vi "FPGA Read Indicator Array Address by Name.vi"(8 "error in (no error)":errorcluster, 9 "Name":string, 10 "Data Type":T1, 11 "FPGA Interface Base in":refnum<class "FPGA Interface Base.lvclass">) -> (0 "error out":errorcluster, 1 "Found?":bool, 2 "Address":u32, 3 "FPGA Interface Base out":refnum<class "FPGA Interface Base.lvclass">, 5 "Num Elements":u32)   [LabVIEW 2010, in "FPGA Interface Base.lvclass"]
uses:
  <userlib>/_FPGA Interface Advanced Tools/FPGA Interface Base/FPGA Interface Base.lvclass
  <vilib>/rvi/DataTransferAndStorage/Container/Common/niFpgaDataTypeControl.ctl
  <userlib>/_FPGA Interface Advanced Tools/FPGA Interface Base/FPGA Interface Base.lvclass/FPGA Interface Base.ctl
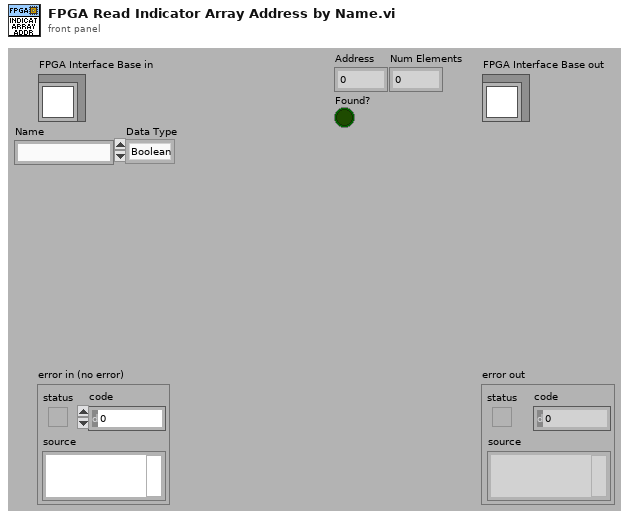
[diagram p1: front panel]
types:
  T1 = typedef "niFpgaDataTypeControl.ctl" = enum32{"Boolean", "I8", "I16", "I32", "I64", "U8", "U16", "U32", "U64", "FXP", "CustomControl"}
  T2 = typedef "FPGA Interface Base.lvclass/FPGA Session.ctl" = refnum<data-value>
  T3 = typedef "FPGA Interface Base.lvclass/FPGA Session Data.ctl" = cluster{"Session Out":u32, "Indicator Scalars":T4, "Indicator Arrays":T6, "Control Scalars":T4, "Control Arrays":T6, "TargetToHost FIFO Channels":T8, "HostToTarget FIFO Channels":T8, "All FIFOs":T9[], "IRQ Context Queue":refnum<queue>}
  T4 = typedef "FPGA Bitfile Utility.lvlib/Scalar Register Set.ctl" = cluster{"Boolean":T5[], "I8":T5[], "I16":T5[], "I32":T5[], "I64":T5[], "U8":T5[], "U16":T5[], "U32":T5[], "U64":T5[]}
  T5 = typedef "FPGA Bitfile Utility.lvlib/Scalar Register.ctl" = cluster{"Address":u32, "Name":string}
  T6 = typedef "FPGA Bitfile Utility.lvlib/Array Register Set.ctl" = cluster{"Boolean":T7[], "I8":T7[], "I16":T7[], "I32":T7[], "I64":T7[], "U8":T7[], "U16":T7[], "U32":T7[], "U64":T7[]}
  T7 = typedef "FPGA Bitfile Utility.lvlib/Array Register.ctl" = cluster{"Address":u32, "Num Elements":u32, "Name":string}
  T8 = typedef "FPGA Bitfile Utility.lvlib/FIFO Channel Set.ctl" = cluster{"Boolean":T9[], "I8":T9[], "I16":T9[], "I32":T9[], "I64":T9[], "U8":T9[], "U16":T9[], "U32":T9[], "U64":T9[]}
  T9 = typedef "FPGA Bitfile Utility.lvlib/FIFO Channel.ctl" = cluster{"Physical Channel":u32, "Name":string}
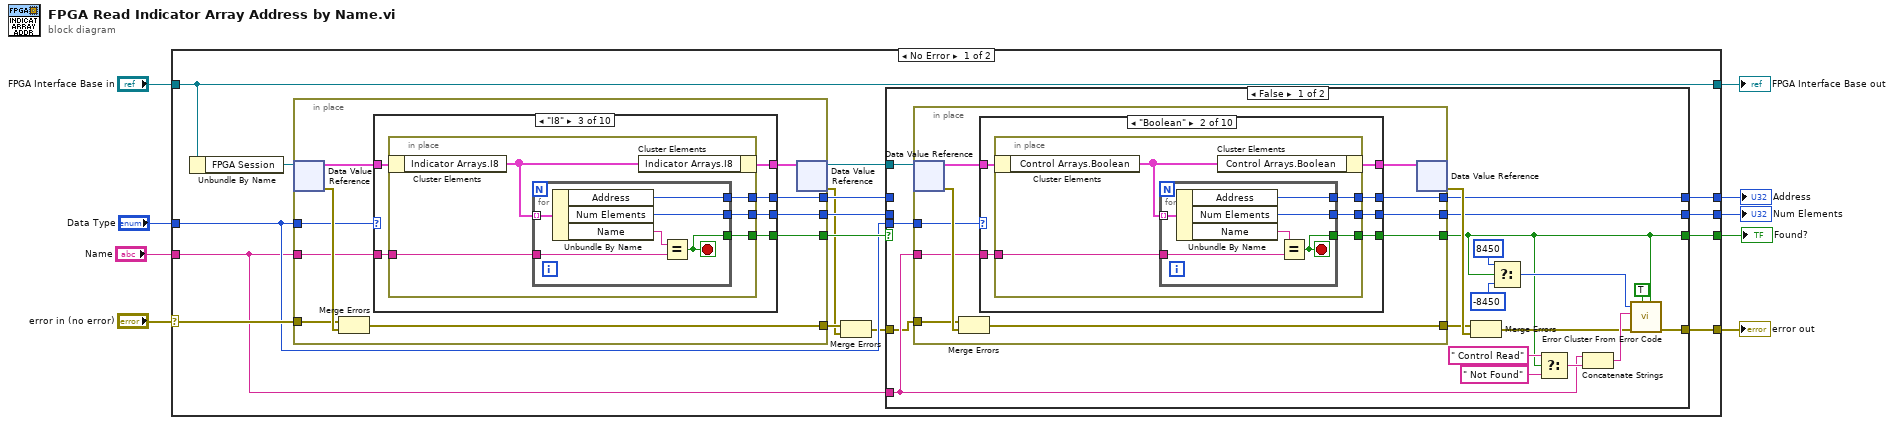
[diagram p0: block diagram]
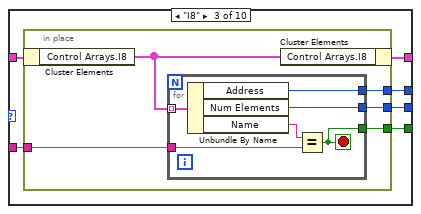
[diagram p3: hidden frame]
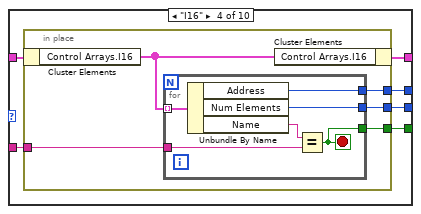
[diagram p4: hidden frame]
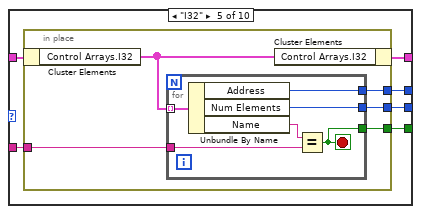
[diagram p5: hidden frame]
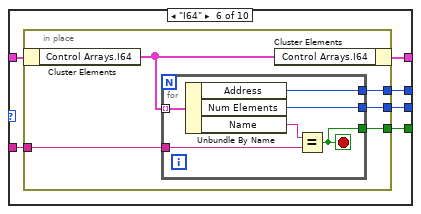
[diagram p6: hidden frame]
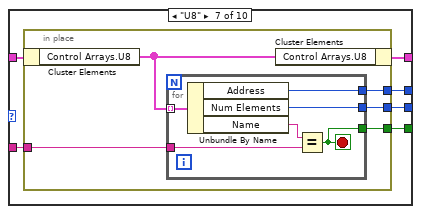
[diagram p7: hidden frame]
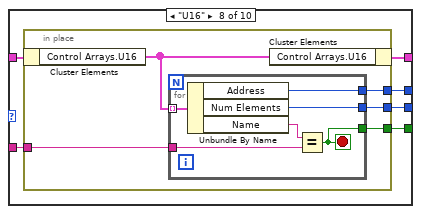
[diagram p8: hidden frame]
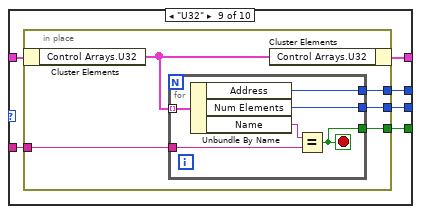
[diagram p9: hidden frame]
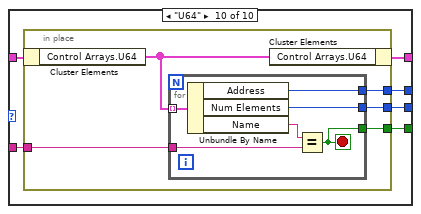
[diagram p10: hidden frame]
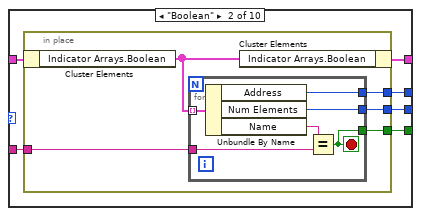
[diagram p13: hidden frame]
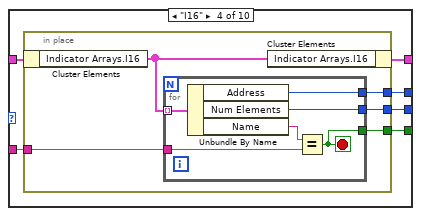
[diagram p14: hidden frame]
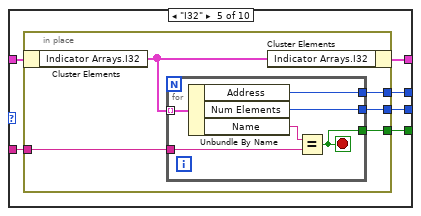
[diagram p15: hidden frame]
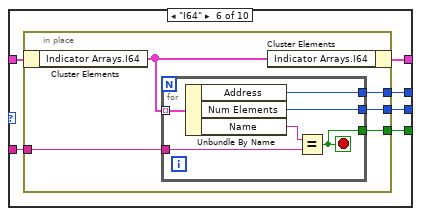
[diagram p16: hidden frame]
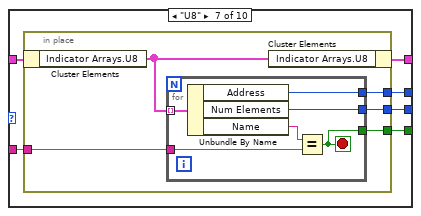
[diagram p17: hidden frame]
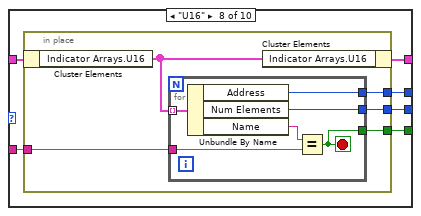
[diagram p18: hidden frame]
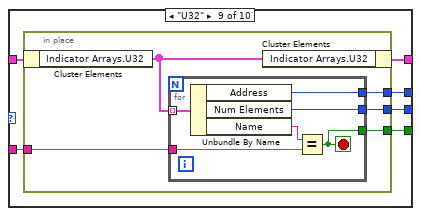
[diagram p19: hidden frame]
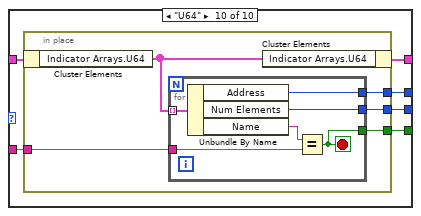
[diagram p20: hidden frame]
diagram:
  n1 = case shown="No Error" "error in (no error)" {
    selector: "error in (no error)" -> [w23 w377]
    tunnel: [w13 w377] -> w8
    tunnel: [w25 w378] -> w6
    tunnel: "FPGA Interface Base in" -> [w25 w378]
    tunnel: [w12 _] -> w5
    tunnel: [w11 _] -> w4
    tunnel: "Name" -> [w14 _]
    tunnel: "Data Type" -> [w18 _]
    tunnel: [w10 _] -> w1
    frame No Error {
      n2 = Unbundle By Name(w25) -> ("FPGA Session"=w24:T2)
      n3 = in-place {
        in-place-border: w14 -> [w219]
        in-place-border: [w218] -> w21
        in-place-border: [w217] -> w19
        in-place-border: [w216] -> w17
        in-place-border: w23 -> [w215]
        in-place-border: w18 -> [w214]
        in-place-border: [w213] -> w20
        n4 = in-place-dvr #1(w24) -> (w221:T3, w222:errorcluster)
        n5 = Merge Errors(w215, w222) -> (w216:errorcluster)
        n6 = case shown="\"I8\"" w214 {
          tunnel: w221 -> [w223 w229 w246 w263 w280 w297 w314 w331 w348 w365]
          tunnel: [w223 w228 w245 w262 w279 w296 w313 w330 w347 w364] -> w220
          tunnel: w219 -> [_ w227 w244 w261 w278 w295 w312 w329 w346 w363]
          tunnel: [_ w226 w243 w260 w277 w294 w311 w328 w345 w362] -> w218
          tunnel: [_ w225 w242 w259 w276 w293 w310 w327 w344 w361] -> w217
          tunnel: [_ w224 w241 w258 w275 w292 w309 w326 w343 w360] -> w213
          frame Default {
          }
          frame "Boolean" {
            n7 = in-place {
              in-place-border: w227 -> [w233]
              in-place-border: [w232] -> w226
              in-place-border: [w231] -> w225
              in-place-border: [w230] -> w224
              n8 = in-place-cluster #2(w229) -> ("Indicator Arrays.Boolean"=w234:T7[])
              n9 = for {
                tunnel: w234 -> [w240] mode=indexing
                tunnel: [w238] -> w232
                tunnel: [w237] -> w231
                tunnel: w233 -> [w236]
                tunnel: [w235] -> w230
                stop <- w237 stop-if-true
                n10 = Unbundle By Name(w240) -> ("Address"=w238:u32, "Num Elements"=w235:u32, "Name"=w239:string)
                n11 = Equal?(x=w239, y=w236) -> (x = y?=w237:bool)
              }
              n12 = in-place-cluster #2("Indicator Arrays.Boolean"=w234) -> (w228:T3)
            }
          }
          frame "I8" {
            n13 = in-place {
              in-place-border: w244 -> [w250]
              in-place-border: [w249] -> w243
              in-place-border: [w248] -> w242
              in-place-border: [w247] -> w241
              n14 = in-place-cluster #3(w246) -> ("Indicator Arrays.I8"=w251:T7[])
              n15 = for {
                tunnel: w251 -> [w257] mode=indexing
                tunnel: [w256] -> w249
                tunnel: [w255] -> w248
                tunnel: w250 -> [w254]
                tunnel: [w252] -> w247
                stop <- w255 stop-if-true
                n16 = Unbundle By Name(w257) -> ("Address"=w256:u32, "Num Elements"=w252:u32, "Name"=w253:string)
                n17 = Equal?(x=w253, y=w254) -> (x = y?=w255:bool)
              }
              n18 = in-place-cluster #3("Indicator Arrays.I8"=w251) -> (w245:T3)
            }
          }
          frame "I16" {
            n19 = in-place {
              in-place-border: w261 -> [w267]
              in-place-border: [w266] -> w260
              in-place-border: [w265] -> w259
              in-place-border: [w264] -> w258
              n20 = in-place-cluster #4(w263) -> ("Indicator Arrays.I16"=w268:T7[])
              n21 = for {
                tunnel: w268 -> [w274] mode=indexing
                tunnel: [w272] -> w266
                tunnel: [w271] -> w265
                tunnel: w267 -> [w270]
                tunnel: [w269] -> w264
                stop <- w271 stop-if-true
                n22 = Unbundle By Name(w274) -> ("Address"=w272:u32, "Num Elements"=w269:u32, "Name"=w273:string)
                n23 = Equal?(x=w273, y=w270) -> (x = y?=w271:bool)
              }
              n24 = in-place-cluster #4("Indicator Arrays.I16"=w268) -> (w262:T3)
            }
          }
          frame "I32" {
            n25 = in-place {
              in-place-border: w278 -> [w284]
              in-place-border: [w283] -> w277
              in-place-border: [w282] -> w276
              in-place-border: [w281] -> w275
              n26 = in-place-cluster #5(w280) -> ("Indicator Arrays.I32"=w285:T7[])
              n27 = for {
                tunnel: w285 -> [w291] mode=indexing
                tunnel: [w289] -> w283
                tunnel: [w288] -> w282
                tunnel: w284 -> [w287]
                tunnel: [w286] -> w281
                stop <- w288 stop-if-true
                n28 = Unbundle By Name(w291) -> ("Address"=w289:u32, "Num Elements"=w286:u32, "Name"=w290:string)
                n29 = Equal?(x=w290, y=w287) -> (x = y?=w288:bool)
              }
              n30 = in-place-cluster #5("Indicator Arrays.I32"=w285) -> (w279:T3)
            }
          }
          frame "I64" {
            n31 = in-place {
              in-place-border: w295 -> [w301]
              in-place-border: [w300] -> w294
              in-place-border: [w299] -> w293
              in-place-border: [w298] -> w292
              n32 = in-place-cluster #6(w297) -> ("Indicator Arrays.I64"=w302:T7[])
              n33 = for {
                tunnel: w302 -> [w308] mode=indexing
                tunnel: [w306] -> w300
                tunnel: [w305] -> w299
                tunnel: w301 -> [w304]
                tunnel: [w303] -> w298
                stop <- w305 stop-if-true
                n34 = Unbundle By Name(w308) -> ("Address"=w306:u32, "Num Elements"=w303:u32, "Name"=w307:string)
                n35 = Equal?(x=w307, y=w304) -> (x = y?=w305:bool)
              }
              n36 = in-place-cluster #6("Indicator Arrays.I64"=w302) -> (w296:T3)
            }
          }
          frame "U8" {
            n37 = in-place {
              in-place-border: w312 -> [w318]
              in-place-border: [w317] -> w311
              in-place-border: [w316] -> w310
              in-place-border: [w315] -> w309
              n38 = in-place-cluster #7(w314) -> ("Indicator Arrays.U8"=w319:T7[])
              n39 = for {
                tunnel: w319 -> [w325] mode=indexing
                tunnel: [w323] -> w317
                tunnel: [w322] -> w316
                tunnel: w318 -> [w321]
                tunnel: [w320] -> w315
                stop <- w322 stop-if-true
                n40 = Unbundle By Name(w325) -> ("Address"=w323:u32, "Num Elements"=w320:u32, "Name"=w324:string)
                n41 = Equal?(x=w324, y=w321) -> (x = y?=w322:bool)
              }
              n42 = in-place-cluster #7("Indicator Arrays.U8"=w319) -> (w313:T3)
            }
          }
          frame "U16" {
            n43 = in-place {
              in-place-border: w329 -> [w335]
              in-place-border: [w334] -> w328
              in-place-border: [w333] -> w327
              in-place-border: [w332] -> w326
              n44 = in-place-cluster #8(w331) -> ("Indicator Arrays.U16"=w336:T7[])
              n45 = for {
                tunnel: w336 -> [w342] mode=indexing
                tunnel: [w340] -> w334
                tunnel: [w339] -> w333
                tunnel: w335 -> [w338]
                tunnel: [w337] -> w332
                stop <- w339 stop-if-true
                n46 = Unbundle By Name(w342) -> ("Address"=w340:u32, "Num Elements"=w337:u32, "Name"=w341:string)
                n47 = Equal?(x=w341, y=w338) -> (x = y?=w339:bool)
              }
              n48 = in-place-cluster #8("Indicator Arrays.U16"=w336) -> (w330:T3)
            }
          }
          frame "U32" {
            n49 = in-place {
              in-place-border: w346 -> [w352]
              in-place-border: [w351] -> w345
              in-place-border: [w350] -> w344
              in-place-border: [w349] -> w343
              n50 = in-place-cluster #9(w348) -> ("Indicator Arrays.U32"=w353:T7[])
              n51 = for {
                tunnel: w353 -> [w359] mode=indexing
                tunnel: [w357] -> w351
                tunnel: [w356] -> w350
                tunnel: w352 -> [w355]
                tunnel: [w354] -> w349
                stop <- w356 stop-if-true
                n52 = Unbundle By Name(w359) -> ("Address"=w357:u32, "Num Elements"=w354:u32, "Name"=w358:string)
                n53 = Equal?(x=w358, y=w355) -> (x = y?=w356:bool)
              }
              n54 = in-place-cluster #9("Indicator Arrays.U32"=w353) -> (w347:T3)
            }
          }
          frame "U64" {
            n55 = in-place {
              in-place-border: w363 -> [w369]
              in-place-border: [w368] -> w362
              in-place-border: [w367] -> w361
              in-place-border: [w366] -> w360
              n56 = in-place-cluster #10(w365) -> ("Indicator Arrays.U64"=w370:T7[])
              n57 = for {
                tunnel: w370 -> [w376] mode=indexing
                tunnel: [w374] -> w368
                tunnel: [w373] -> w367
                tunnel: w369 -> [w372]
                tunnel: [w371] -> w366
                stop <- w373 stop-if-true
                n58 = Unbundle By Name(w376) -> ("Address"=w374:u32, "Num Elements"=w371:u32, "Name"=w375:string)
                n59 = Equal?(x=w375, y=w372) -> (x = y?=w373:bool)
              }
              n60 = in-place-cluster #10("Indicator Arrays.U64"=w370) -> (w364:T3)
            }
          }
        }
        n61 = in-place-dvr #1(w220) -> (w22:T2, w15:errorcluster)
      }
      n62 = Merge Errors(w17, w15) -> (w16:errorcluster)
      n63 = case shown="False" w19 {
        selector: w19 -> [_ w211]
        tunnel: w22 -> [w34 _]
        tunnel: w16 -> [w29 w210]
        tunnel: w21 -> [_ w212]
        tunnel: [w32 w212] -> w12
        tunnel: [w27 w211] -> w11
        tunnel: [w36 w210] -> w13
        tunnel: w14 -> [w30 _]
        tunnel: w18 -> [w31 _]
        tunnel: w20 -> [_ w209]
        tunnel: [w26 w209] -> w10
        frame False {
          n64 = in-place {
            in-place-border: w30 -> [w48]
            in-place-border: [w49] -> w32
            in-place-border: [w46] -> w27
            in-place-border: [w53] -> w28
            in-place-border: w29 -> [w52]
            in-place-border: w31 -> [w47]
            in-place-border: [w45] -> w26
            n65 = in-place-dvr #11(w34) -> (w51:T3, w54:errorcluster)
            n66 = Merge Errors(w52, w54) -> (w53:errorcluster)
            n67 = case shown="\"Boolean\"" w47 {
              tunnel: w51 -> [w55 w61 w78 w95 w112 w129 w146 w163 w180 w197]
              tunnel: [w55 w60 w77 w94 w111 w128 w145 w162 w179 w196] -> w50
              tunnel: w48 -> [_ w59 w76 w93 w110 w127 w144 w161 w178 w195]
              tunnel: [_ w58 w75 w92 w109 w126 w143 w160 w177 w194] -> w49
              tunnel: [_ w57 w74 w91 w108 w125 w142 w159 w176 w193] -> w46
              tunnel: [_ w56 w73 w90 w107 w124 w141 w158 w175 w192] -> w45
              frame Default {
              }
              frame "Boolean" {
                n68 = in-place {
                  in-place-border: w59 -> [w65]
                  in-place-border: [w64] -> w58
                  in-place-border: [w63] -> w57
                  in-place-border: [w62] -> w56
                  n69 = in-place-cluster #12(w61) -> ("Control Arrays.Boolean"=w66:T7[])
                  n70 = for {
                    tunnel: w66 -> [w72] mode=indexing
                    tunnel: [w70] -> w64
                    tunnel: [w69] -> w63
                    tunnel: w65 -> [w68]
                    tunnel: [w67] -> w62
                    stop <- w69 stop-if-true
                    n71 = Unbundle By Name(w72) -> ("Address"=w70:u32, "Num Elements"=w67:u32, "Name"=w71:string)
                    n72 = Equal?(x=w71, y=w68) -> (x = y?=w69:bool)
                  }
                  n73 = in-place-cluster #12("Control Arrays.Boolean"=w66) -> (w60:T3)
                }
              }
              frame "I8" {
                n74 = in-place {
                  in-place-border: w76 -> [w82]
                  in-place-border: [w81] -> w75
                  in-place-border: [w80] -> w74
                  in-place-border: [w79] -> w73
                  n75 = in-place-cluster #13(w78) -> ("Control Arrays.I8"=w83:T7[])
                  n76 = for {
                    tunnel: w83 -> [w89] mode=indexing
                    tunnel: [w88] -> w81
                    tunnel: [w87] -> w80
                    tunnel: w82 -> [w86]
                    tunnel: [w84] -> w79
                    stop <- w87 stop-if-true
                    n77 = Unbundle By Name(w89) -> ("Address"=w88:u32, "Num Elements"=w84:u32, "Name"=w85:string)
                    n78 = Equal?(x=w85, y=w86) -> (x = y?=w87:bool)
                  }
                  n79 = in-place-cluster #13("Control Arrays.I8"=w83) -> (w77:T3)
                }
              }
              frame "I16" {
                n80 = in-place {
                  in-place-border: w93 -> [w99]
                  in-place-border: [w98] -> w92
                  in-place-border: [w97] -> w91
                  in-place-border: [w96] -> w90
                  n81 = in-place-cluster #14(w95) -> ("Control Arrays.I16"=w100:T7[])
                  n82 = for {
                    tunnel: w100 -> [w106] mode=indexing
                    tunnel: [w104] -> w98
                    tunnel: [w103] -> w97
                    tunnel: w99 -> [w102]
                    tunnel: [w101] -> w96
                    stop <- w103 stop-if-true
                    n83 = Unbundle By Name(w106) -> ("Address"=w104:u32, "Num Elements"=w101:u32, "Name"=w105:string)
                    n84 = Equal?(x=w105, y=w102) -> (x = y?=w103:bool)
                  }
                  n85 = in-place-cluster #14("Control Arrays.I16"=w100) -> (w94:T3)
                }
              }
              frame "I32" {
                n86 = in-place {
                  in-place-border: w110 -> [w116]
                  in-place-border: [w115] -> w109
                  in-place-border: [w114] -> w108
                  in-place-border: [w113] -> w107
                  n87 = in-place-cluster #15(w112) -> ("Control Arrays.I32"=w117:T7[])
                  n88 = for {
                    tunnel: w117 -> [w123] mode=indexing
                    tunnel: [w121] -> w115
                    tunnel: [w120] -> w114
                    tunnel: w116 -> [w119]
                    tunnel: [w118] -> w113
                    stop <- w120 stop-if-true
                    n89 = Unbundle By Name(w123) -> ("Address"=w121:u32, "Num Elements"=w118:u32, "Name"=w122:string)
                    n90 = Equal?(x=w122, y=w119) -> (x = y?=w120:bool)
                  }
                  n91 = in-place-cluster #15("Control Arrays.I32"=w117) -> (w111:T3)
                }
              }
              frame "I64" {
                n92 = in-place {
                  in-place-border: w127 -> [w133]
                  in-place-border: [w132] -> w126
                  in-place-border: [w131] -> w125
                  in-place-border: [w130] -> w124
                  n93 = in-place-cluster #16(w129) -> ("Control Arrays.I64"=w134:T7[])
                  n94 = for {
                    tunnel: w134 -> [w140] mode=indexing
                    tunnel: [w138] -> w132
                    tunnel: [w137] -> w131
                    tunnel: w133 -> [w136]
                    tunnel: [w135] -> w130
                    stop <- w137 stop-if-true
                    n95 = Unbundle By Name(w140) -> ("Address"=w138:u32, "Num Elements"=w135:u32, "Name"=w139:string)
                    n96 = Equal?(x=w139, y=w136) -> (x = y?=w137:bool)
                  }
                  n97 = in-place-cluster #16("Control Arrays.I64"=w134) -> (w128:T3)
                }
              }
              frame "U8" {
                n98 = in-place {
                  in-place-border: w144 -> [w150]
                  in-place-border: [w149] -> w143
                  in-place-border: [w148] -> w142
                  in-place-border: [w147] -> w141
                  n99 = in-place-cluster #17(w146) -> ("Control Arrays.U8"=w151:T7[])
                  n100 = for {
                    tunnel: w151 -> [w157] mode=indexing
                    tunnel: [w155] -> w149
                    tunnel: [w154] -> w148
                    tunnel: w150 -> [w153]
                    tunnel: [w152] -> w147
                    stop <- w154 stop-if-true
                    n101 = Unbundle By Name(w157) -> ("Address"=w155:u32, "Num Elements"=w152:u32, "Name"=w156:string)
                    n102 = Equal?(x=w156, y=w153) -> (x = y?=w154:bool)
                  }
                  n103 = in-place-cluster #17("Control Arrays.U8"=w151) -> (w145:T3)
                }
              }
              frame "U16" {
                n104 = in-place {
                  in-place-border: w161 -> [w167]
                  in-place-border: [w166] -> w160
                  in-place-border: [w165] -> w159
                  in-place-border: [w164] -> w158
                  n105 = in-place-cluster #18(w163) -> ("Control Arrays.U16"=w168:T7[])
                  n106 = for {
                    tunnel: w168 -> [w174] mode=indexing
                    tunnel: [w172] -> w166
                    tunnel: [w171] -> w165
                    tunnel: w167 -> [w170]
                    tunnel: [w169] -> w164
                    stop <- w171 stop-if-true
                    n107 = Unbundle By Name(w174) -> ("Address"=w172:u32, "Num Elements"=w169:u32, "Name"=w173:string)
                    n108 = Equal?(x=w173, y=w170) -> (x = y?=w171:bool)
                  }
                  n109 = in-place-cluster #18("Control Arrays.U16"=w168) -> (w162:T3)
                }
              }
              frame "U32" {
                n110 = in-place {
                  in-place-border: w178 -> [w184]
                  in-place-border: [w183] -> w177
                  in-place-border: [w182] -> w176
                  in-place-border: [w181] -> w175
                  n111 = in-place-cluster #19(w180) -> ("Control Arrays.U32"=w185:T7[])
                  n112 = for {
                    tunnel: w185 -> [w191] mode=indexing
                    tunnel: [w189] -> w183
                    tunnel: [w188] -> w182
                    tunnel: w184 -> [w187]
                    tunnel: [w186] -> w181
                    stop <- w188 stop-if-true
                    n113 = Unbundle By Name(w191) -> ("Address"=w189:u32, "Num Elements"=w186:u32, "Name"=w190:string)
                    n114 = Equal?(x=w190, y=w187) -> (x = y?=w188:bool)
                  }
                  n115 = in-place-cluster #19("Control Arrays.U32"=w185) -> (w179:T3)
                }
              }
              frame "U64" {
                n116 = in-place {
                  in-place-border: w195 -> [w201]
                  in-place-border: [w200] -> w194
                  in-place-border: [w199] -> w193
                  in-place-border: [w198] -> w192
                  n117 = in-place-cluster #20(w197) -> ("Control Arrays.U64"=w202:T7[])
                  n118 = for {
                    tunnel: w202 -> [w208] mode=indexing
                    tunnel: [w206] -> w200
                    tunnel: [w205] -> w199
                    tunnel: w201 -> [w204]
                    tunnel: [w203] -> w198
                    stop <- w205 stop-if-true
                    n119 = Unbundle By Name(w208) -> ("Address"=w206:u32, "Num Elements"=w203:u32, "Name"=w207:string)
                    n120 = Equal?(x=w207, y=w204) -> (x = y?=w205:bool)
                  }
                  n121 = in-place-cluster #20("Control Arrays.U64"=w202) -> (w196:T3)
                }
              }
            }
            n122 = in-place-dvr #11(w50) -> (w33:errorcluster)  [unwired: 1 out]
          }
          n123 = Merge Errors(w28, w33) -> (w37:errorcluster)
          n124 = Select(t=8450 ("error code (0)"), s=w27, f=-8450 ("error code (0)")) -> (s? t:f=w35:i32)
          n125 = Select(t=" Control Read" ("string"), s=w27, f=" Not Found" ("string")) -> (s? t:f=w40:string)
          n126 = Concatenate Strings(w30, w40) -> (w38:string)
          n127 = call <vilib>:"Error Cluster From Error Code.vi"("is warning? (False)"=w27, "show call chain? (False)"=TRUE, "error in (no error)"=w37, "error message (\"\")"=w38, "error code (0)"=w35) -> ("error out"=w36:errorcluster)  [unwired: 4 in]
        }
        frame True {
        }
      }
    }
    frame Error {
    }
  }
  "error out" <- w8
  "FPGA Interface Base out" <- w6
  "Address" <- w5
  "Found?" <- w4
  "Num Elements" <- w1
